vi "Resample.vi"(8 "error in (no error)":errorcluster, 11 "Instrument.DAQ":refnum<class "Instrument.DAQ.lvclass">) -> (0 "error out":errorcluster, 3 "Instrument.DAQ out":refnum<class "Instrument.DAQ.lvclass">)   [LabVIEW 2019, in "Instrument.Lockin.lvlib" / "Instrument.DAQ.lvclass"]
uses:
  Instrument.DAQ.lvclass
  Instrument.DAQ.lvclass/Instrument.DAQ.ctl
  <vilib>/measure/NI_MAPro.lvlib
  <vilib>/Analysis/NI_AALPro.lvlib
  <vilib>/Analysis/2dsp.llb/Decimate (single shot, DBL).vi
  <vilib>/measure/maresamp.llb/Resample N Waveforms (continuous).vi
  <vilib>/Analysis/2dsp.llb/Rational Resample (single channel, DBL).vi
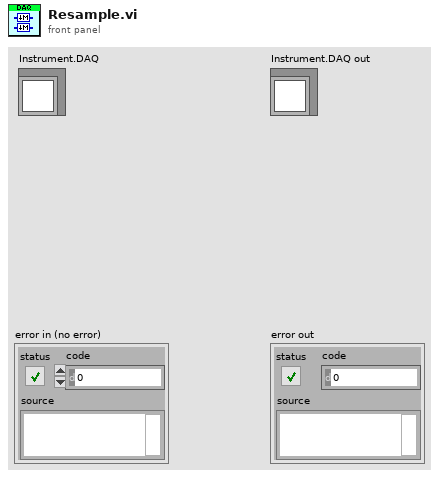
[diagram p1: front panel]
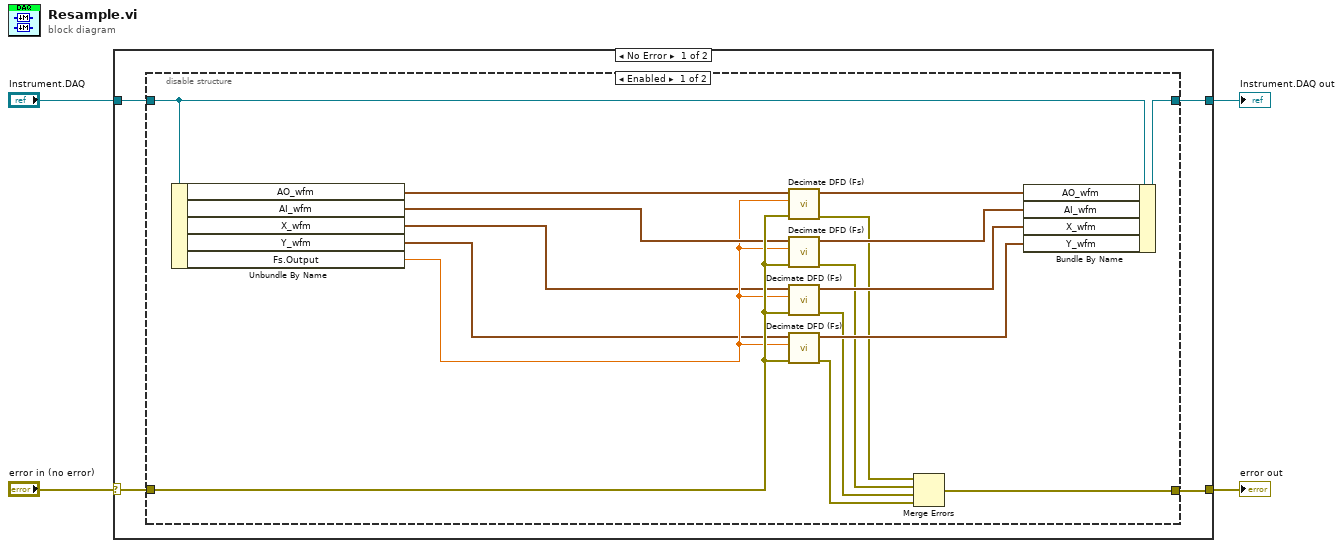
[diagram p0: block diagram]
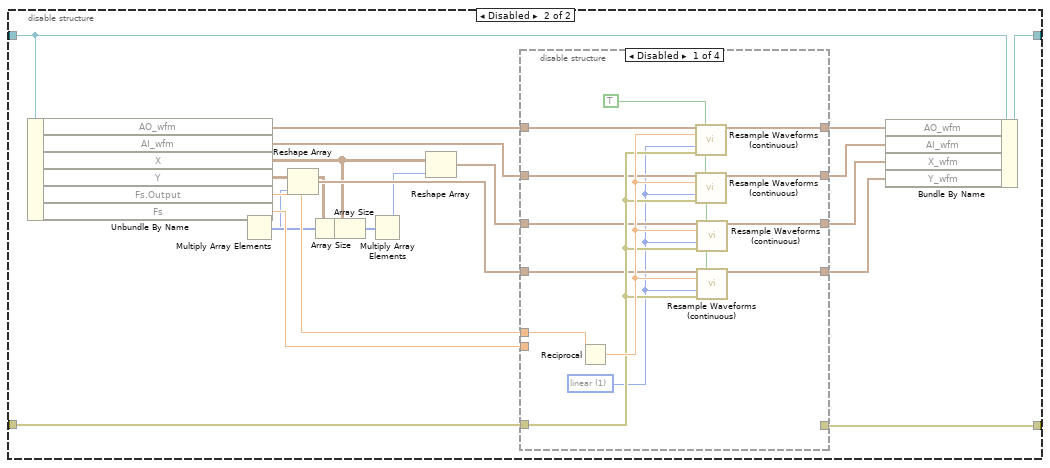
[diagram p2: hidden frame]
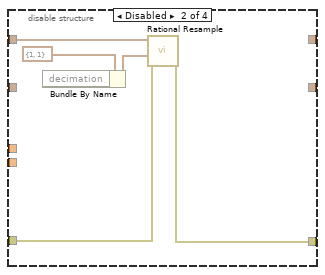
[diagram p3: hidden frame]
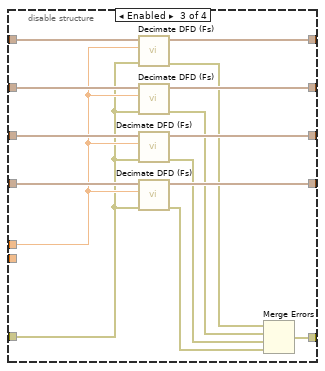
[diagram p4: hidden frame]
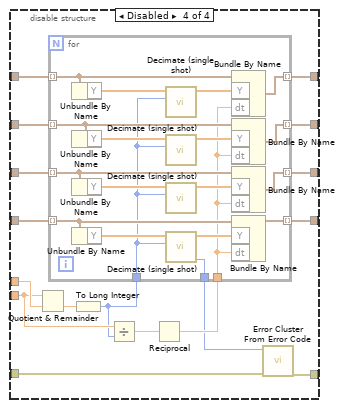
[diagram p5: hidden frame]
diagram:
  n1 = case shown="No Error" "error in (no error)" {
    selector: "error in (no error)" -> [w8 w120]
    tunnel: [w6 w120] -> w3
    tunnel: "Instrument.DAQ" -> [w7 w119]
    tunnel: [w5 w119] -> w1
    frame No Error {
      n2 = disable-structure shown="Enabled" {
        disable-tunnel: w8 -> [w25 w45]
        disable-tunnel: w7 -> [w22 w42]
        disable-tunnel: [w17 w36] -> w6
        disable-tunnel: [w13 w26] -> w5
        frame Enabled {
          n3 = Unbundle By Name(w22) -> ("AO_wfm"=w24:waveform(dbl)[], "AI_wfm"=w23:waveform(dbl)[], "X_wfm"=w14:waveform(dbl)[], "Y_wfm"=w15:waveform(dbl)[], "Fs.Output"=w16:dbl)
          n4 = call "Decimate DFD (Fs).vi"("error in (no error)"=w25, "output fs[Hz]"=w16, "Waveforms in"=w24) -> ("error out"=w12:errorcluster, "waveforms out"=w21:waveform(dbl)[])  [unwired: 7 in]
          n5 = call "Decimate DFD (Fs).vi"("error in (no error)"=w25, "output fs[Hz]"=w16, "Waveforms in"=w23) -> ("error out"=w11:errorcluster, "waveforms out"=w20:waveform(dbl)[])  [unwired: 7 in]
          n6 = call "Decimate DFD (Fs).vi"("error in (no error)"=w25, "output fs[Hz]"=w16, "Waveforms in"=w14) -> ("error out"=w10:errorcluster, "waveforms out"=w19:waveform(dbl)[])  [unwired: 7 in]
          n7 = call "Decimate DFD (Fs).vi"("error in (no error)"=w25, "output fs[Hz]"=w16, "Waveforms in"=w15) -> ("error out"=w9:errorcluster, "waveforms out"=w18:waveform(dbl)[])  [unwired: 7 in]
          n8 = Merge Errors(w12, w11, w10, w9) -> (w17:errorcluster)
          n9 = Bundle By Name(cluster=w22, "AO_wfm"=w21, "AI_wfm"=w20, "X_wfm"=w19, "Y_wfm"=w18) -> (w13:refnum<class "Instrument.DAQ.lvclass">)
        }
        frame Disabled {
          n10 = Unbundle By Name(w42) -> ("AO_wfm"=w44:waveform(dbl)[], "AI_wfm"=w43:waveform(dbl)[], "X"=w28:waveform(dbl)[][], "Y"=w32:waveform(dbl)[][], "Fs.Output"=w33:dbl, "Fs"=w37:dbl)
          n11 = Array Size(array=w32) -> (size(s)=w31:i32[])
          n12 = Multiply Array Elements(1:w31) -> (0:w30:i32)
          n13 = Reshape Array(w32, w30) -> (w34:waveform(dbl)[])
          n14 = Array Size(array=w28) -> (size(s)=w29:i32[])
          n15 = Multiply Array Elements(1:w29) -> (0:w27:i32)
          n16 = Reshape Array(w28, w27) -> (w35:waveform(dbl)[])
          n17 = disable-structure shown="Disabled" {
            disable-tunnel: w45 -> [w61 w64 w75 w84]
            disable-tunnel: w33 -> [w56 _ w76 w99]
            disable-tunnel: [w55 _ w79 w93] -> w41
            disable-tunnel: [w54 _ w80 w91] -> w40
            disable-tunnel: [w53 _ w73 w92] -> w39
            disable-tunnel: [w52 _ w74 w90] -> w38
            disable-tunnel: w44 -> [w51 _ w82 w96]
            disable-tunnel: w43 -> [w50 _ w81 w95]
            disable-tunnel: w34 -> [w49 _ w77 w97]
            disable-tunnel: w35 -> [w48 w67 w78 w98]
            disable-tunnel: w37 -> [_ _ _ w89]
            disable-tunnel: [_ w63 w68 w83] -> w36
            frame Disabled {
              w46 = TRUE ("reset")
              w47 = u16 1 items=["coerce", "linear", "spline", "FIR filter"] ("interpolation mode")
              n18 = Reciprocal(x=w56) -> (1/x=w62:dbl)
              n19 = call-poly <vilib>:"Resample Waveforms (continuous).vi"("waveforms in"=w51, "reset"=w46, "dt"=w62, "interpolation mode"=w47, "error in (no error)"=w61) -> ("resampled waveforms out"=w55:waveform(dbl)[], "error out"=w57:errorcluster)  [unwired: 6 in, 3 out]
              n20 = call-poly <vilib>:"Resample Waveforms (continuous).vi"("waveforms in"=w50, "reset"=w46, "dt"=w62, "interpolation mode"=w47, "error in (no error)"=w61) -> ("resampled waveforms out"=w54:waveform(dbl)[], "error out"=w58:errorcluster)  [unwired: 6 in, 3 out]
              n21 = call-poly <vilib>:"Resample Waveforms (continuous).vi"("waveforms in"=w48, "reset"=w46, "dt"=w62, "interpolation mode"=w47, "error in (no error)"=w61) -> ("resampled waveforms out"=w53:waveform(dbl)[], "error out"=w59:errorcluster)  [unwired: 6 in, 3 out]
              n22 = call-poly <vilib>:"Resample Waveforms (continuous).vi"("waveforms in"=w49, "reset"=w46, "dt"=w62, "interpolation mode"=w47, "error in (no error)"=w61) -> ("resampled waveforms out"=w52:waveform(dbl)[], "error out"=w60:errorcluster)  [unwired: 6 in, 3 out]
            }
            frame Disabled {
              n23 = Bundle By Name(cluster=cluster{"interpolation":i32, "decimation":i32} {"interpolation"=1, "decimation"=1} ("resample factor")) -> (w65:cluster{"interpolation":i32, "decimation":i32})  [unwired: 1 in]
              n24 = call-poly <vilib>:"Rational Resample.vi"("error in (no error)"=w64, "resample factor"=w65, "X"=w67) -> ("error out"=w63:errorcluster)  [unwired: 6 in, 2 out]
            }
            frame Enabled {
              n25 = call "Decimate DFD (Fs).vi"("error in (no error)"=w75, "output fs[Hz]"=w76, "Waveforms in"=w82) -> ("error out"=w72:errorcluster, "waveforms out"=w79:waveform(dbl)[])  [unwired: 7 in]
              n26 = call "Decimate DFD (Fs).vi"("error in (no error)"=w75, "output fs[Hz]"=w76, "Waveforms in"=w81) -> ("error out"=w71:errorcluster, "waveforms out"=w80:waveform(dbl)[])  [unwired: 7 in]
              n27 = call "Decimate DFD (Fs).vi"("error in (no error)"=w75, "output fs[Hz]"=w76, "Waveforms in"=w78) -> ("error out"=w70:errorcluster, "waveforms out"=w73:waveform(dbl)[])  [unwired: 7 in]
              n28 = call "Decimate DFD (Fs).vi"("error in (no error)"=w75, "output fs[Hz]"=w76, "Waveforms in"=w77) -> ("error out"=w69:errorcluster, "waveforms out"=w74:waveform(dbl)[])  [unwired: 7 in]
              n29 = Merge Errors(w72, w71, w70, w69) -> (w68:errorcluster)
            }
            frame Disabled {
              n30 = Quotient & Remainder(x=w89, y=w99) -> (floor(x/y)=w94:dbl)  [unwired: 1 out]
              n31 = To Long Integer(number=w94) -> (32bit integer=w88:i32)
              n32 = Divide(x=w89, y=w88) -> (x/y=w87:dbl)
              n33 = Reciprocal(x=w87) -> (1/x=w86:dbl)
              n34 = for {
                tunnel: w98 -> [w107] mode=indexing
                tunnel: w97 -> [w103] mode=indexing
                tunnel: w96 -> [w109] mode=indexing
                tunnel: w95 -> [w108] mode=indexing
                tunnel: w88 -> [w102]
                tunnel: [w117] -> w93 mode=indexing
                tunnel: [w113] -> w92 mode=indexing
                tunnel: [w112] -> w91 mode=indexing
                tunnel: [w111] -> w90 mode=indexing
                tunnel: w86 -> [w101]
                tunnel: [w100] -> w85
                n35 = Unbundle By Name(w109) -> ("Y"=w110:dbl[])
                n36 = Unbundle By Name(w108) -> ("Y"=w105:dbl[])
                n37 = Unbundle By Name(w107) -> ("Y"=w106:dbl[])
                n38 = Unbundle By Name(w103) -> ("Y"=w104:dbl[])
                n39 = call-poly <vilib>:"Decimate (single shot).vi"("decimating factor"=w102, "X"=w110) -> ("Decimated Array"=w118:dbl[])  [unwired: 8 in, 1 out]
                n40 = call-poly <vilib>:"Decimate (single shot).vi"("decimating factor"=w102, "X"=w105) -> ("Decimated Array"=w115:dbl[])  [unwired: 8 in, 1 out]
                n41 = call-poly <vilib>:"Decimate (single shot).vi"("decimating factor"=w102, "X"=w106) -> ("Decimated Array"=w114:dbl[])  [unwired: 8 in, 1 out]
                n42 = call-poly <vilib>:"Decimate (single shot).vi"("decimating factor"=w102, "X"=w104) -> ("error"=w100:i32, "Decimated Array"=w116:dbl[])  [unwired: 8 in]
                n43 = Bundle By Name(cluster=w109, "Y"=w118, "dt"=w101) -> (w117:waveform(dbl))
                n44 = Bundle By Name(cluster=w108, "Y"=w115, "dt"=w101) -> (w112:waveform(dbl))
                n45 = Bundle By Name(cluster=w107, "Y"=w114, "dt"=w101) -> (w113:waveform(dbl))
                n46 = Bundle By Name(cluster=w103, "Y"=w116, "dt"=w101) -> (w111:waveform(dbl))
              }
              n47 = call <vilib>:"Error Cluster From Error Code.vi"("error in (no error)"=w84, "error code (0)"=w85) -> ("error out"=w83:errorcluster)  [unwired: 7 in]
            }
          }
          n48 = Bundle By Name(cluster=w42, "AO_wfm"=w41, "AI_wfm"=w40, "X_wfm"=w39, "Y_wfm"=w38) -> (w26:refnum<class "Instrument.DAQ.lvclass">)
        }
      }
    }
    frame Error {
    }
  }
  "error out" <- w3
  "Instrument.DAQ out" <- w1
